vi "X Array Index to Range.vi"(2 "X Range (index)":i32=1, 3 "X-array":dbl[](array[numeric])) -> (0 "X Range":dbl)   [LabVIEW 2019, in "xy_utilities.lvlib"]
uses:
  xy_utilities.lvlib
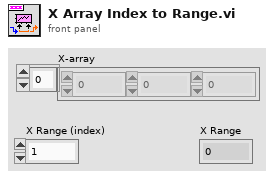
[diagram p1: front panel]
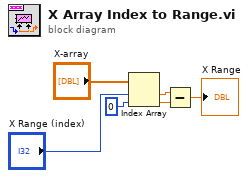
[diagram p0: block diagram]
diagram:
  n1 = Index Array(array="X-array", index #1="X Range (index)", index #2=0 ("index")) -> (element #1=w3:dbl, element #2=w2:dbl)
  n2 = Subtract(x=w3, y=w2) -> (x-y=→"X Range":dbl)
